vi "SENS_FREQ_CENT.vi"(0 "VISA IN":refnum<visa-resource-name>, 1 "Center Frq.":dbl, 5 "error in":errorcluster, 7 "Channel":i32) -> (14 "VISA Out":refnum<visa-resource-name>, 19 "error out":errorcluster)   [LabVIEW 2018, in "PNA-X.lvlib"]
doc: "SENSe<cnum>:FREQuency:CENTer <num> \n(Read-Write) Sets the center frequency of the analyzer. \nParameters \n<cnum> Any existing channel number. If unspecified, value is set to 1 \n<num> Center frequency. Choose any number between the minimum and maximum \nfrequency limits of the analyzer. Units are Hz. \nSee Note \nExamples SENS:FREQ:CENT 1000000 \nsense2:frequency:center 1mhz \nsense2:frequency:center 1e6 \nQuery Syntax SENSe<cnum>:FREQuency:CENTer? \nReturn Type Numeric \nDefault Center of the analyzer's frequency span \n1744"
uses:
  PNA-X.lvlib
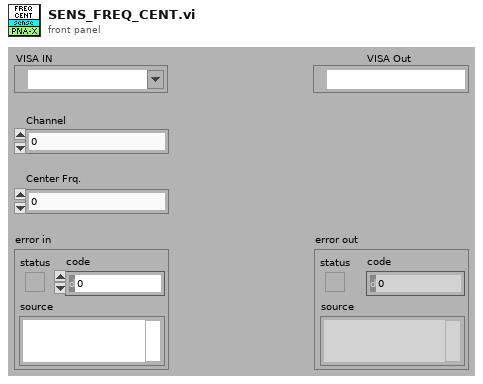
[diagram p1: front panel]
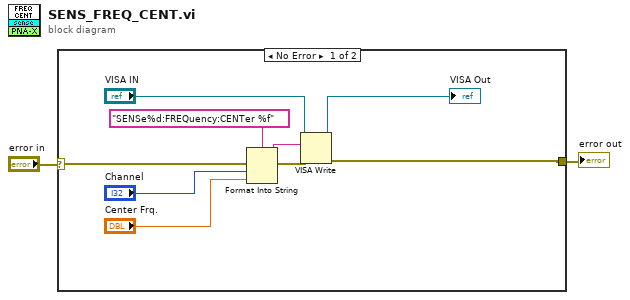
[diagram p0: block diagram]
diagram:
  n1 = case shown="No Error" "error in" {
    selector: "error in" -> [w11 w12]
    tunnel: [w6 w12] -> w1
    frame No Error {
      n2 = Format Into String(format string="SENSe%d:FREQuency:CENTer %f" ("Cmdline"), error in=w11, "Channel", "Center Frq.") -> (resulting string=w9:string, error out=w10:errorcluster)  [unwired: 1 in]
      n3 = VISA Write(VISA resource name="VISA IN", write buffer=w9, error in (no error)=w10) -> (VISA resource name out=→"VISA Out":refnum<visa-resource-name>, error out=w6:errorcluster)  [unwired: 1 out]
    }
    frame Error {
    }
  }
  "error out" <- w1
